vi "Format Channel Configuration Log.vi"(8 "error in (no error)":errorcluster, 10 "Channel Type (ao/ai)":enum16{"ao", "ai"}(ring), 11 "Instrument.Lockin in":refnum<class "Instrument.Lockin.lvclass">) -> (0 "error out":errorcluster, 1 "Channel Configuration":T1[](array[typedef]), 2 "Log Paths":string, 3 "Instrument.Lockin out":refnum<class "Instrument.Lockin.lvclass">, 4 "Times":timestamp[](array[timestamp]))   [LabVIEW 2019, in "Instrument.Lockin.lvlib" / "Instrument.Lockin.lvclass"]
uses:
  Instrument.Lockin.lvclass
  Typedefs/Lockin.LogConfiguration.Channels--Cluster.ctl
  Instrument.Lockin.lvclass/Instrument.Lockin.ctl
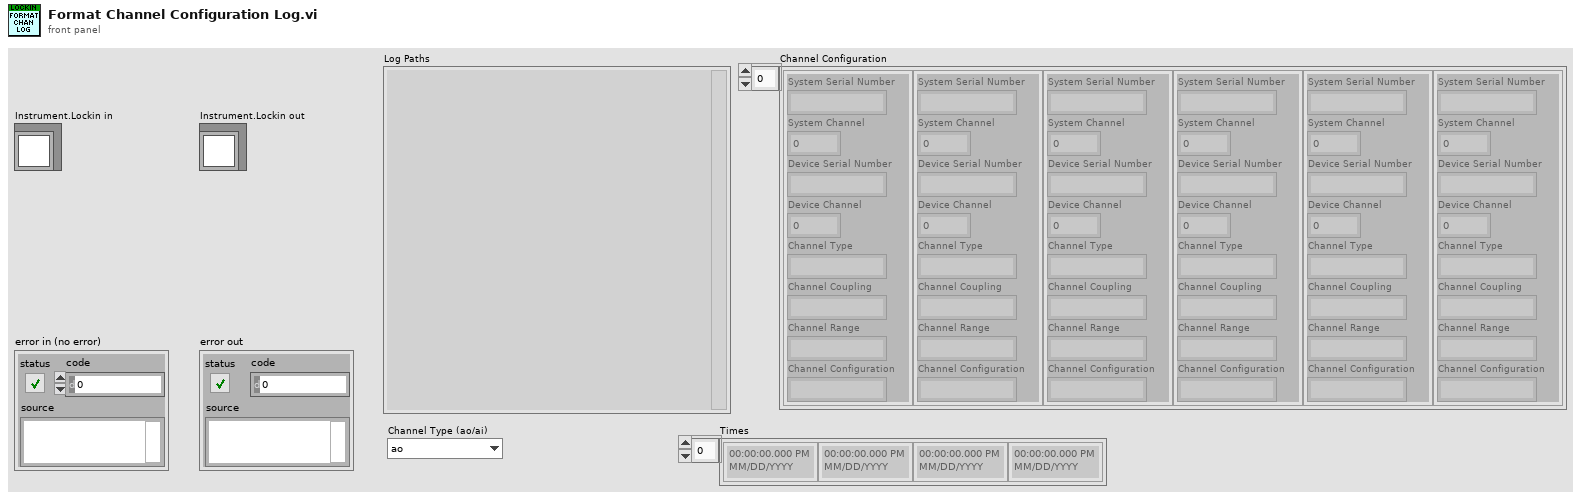
[diagram p1: front panel]
types:
  T1 = typedef "Instrument.Lockin.lvlib/Instrument.Lockin.lvclass/Lockin.LogConfiguration.Channels--Cluster.ctl" = cluster{"System Serial Number":string, "System Channel":i32, "Device Serial Number":string, "Device Channel":i32, "Channel Type":string, "Channel Coupling":string, "Channel Range":string, "Channel Configuration":string}
  T2 = typedef "Instrument.Lockin.lvlib/Instrument.DAQ.lvclass/AO.Channel--Cluster--Array.ctl" = T3[]
  T3 = typedef "Instrument.Lockin.lvlib/Instrument.DAQ.lvclass/AO.Channel--Cluster.ctl" = cluster{"Enable?":bool, "Channel":i32, "Amplitude":dbl, "Offset":dbl, "Frequency":dbl, "Phase":dbl, "Function":T4, "Sweeping?":bool, "Limit AC":bool, "Limit DC?":bool, "Duty Cycle":bool}
  T4 = typedef "Instrument.Lockin.lvlib/Instrument.DAQ.lvclass/AO.Channel.Function--Enum.ctl" = enum16{"sine", "square", "triangle", "saw"}
  T5 = typedef "Instrument.Lockin.lvlib/Instrument.DAQ.lvclass/DeviceInfo--Cluster.ctl" = cluster{"DeviceName":string, "DevIsSimulated":bool, "DeviceSerialNumber":string, "ProductType":string, "ProductCategory":i32, "ProductNumber":u32, "ChassisNumber":u32, "SlotNumber":u32, "ChassisName":string, "ChassisSerialNumber":string, "DevTemp":dbl, "SelfCal.LastDate/Time":string, "SelfCal.LastTemp":dbl, "calibration due?":bool}
  T6 = typedef "Instrument.Lockin.lvlib/Instrument.DAQ.lvclass/DAQ.Config.AO--Cluster--Array.ctl" = cluster{"Channels":tag, "Range":T7, "terminal configuration":T8, "Type":T9}[]
  T7 = typedef "Instrument.Lockin.lvlib/Instrument.DAQ.lvclass/DAQ.Config.AO.Range--enum.ctl" = enum16{"±0.1", "±1.0", "±10.0", ""}
  T8 = typedef "Instrument.Lockin.lvlib/Instrument.DAQ.lvclass/DAQ.TerminalConfiguration--ring.ctl" = i32
  T9 = typedef "Instrument.Lockin.lvlib/Instrument.DAQ.lvclass/DAQ.Type--enum.ctl" = enum16{"None", "USB-4431", "PXI-446x"}
  T10 = typedef "Instrument.Lockin.lvlib/Instrument.DAQ.lvclass/AI.Channel--Cluster--Array.ctl" = T11[]
  T11 = typedef "Instrument.Lockin.lvlib/Instrument.DAQ.lvclass/AI.Channel--Cluster.ctl" = cluster{"Enable?":bool, "Channel":i32, "References":u16[], "reference index":i32}
  T12 = typedef "Instrument.Lockin.lvlib/Instrument.DAQ.lvclass/DAQ.Config.AI--Cluster--Array.ctl" = cluster{"Channels":tag, "Coupling":T13, "Range":T14, "terminal configuration":T8, "Type":T9}[]
  T13 = typedef "Instrument.Lockin.lvlib/Instrument.DAQ.lvclass/DAQ.Config.AI.Coupling--enum.ctl" = u16
  T14 = typedef "Instrument.Lockin.lvlib/Instrument.DAQ.lvclass/DAQ.Config.AI.Range--enum.ctl" = enum16{"±0.316", "±1.00", "±3.16", "±10.0", "±31.6", "±42.4", ""}
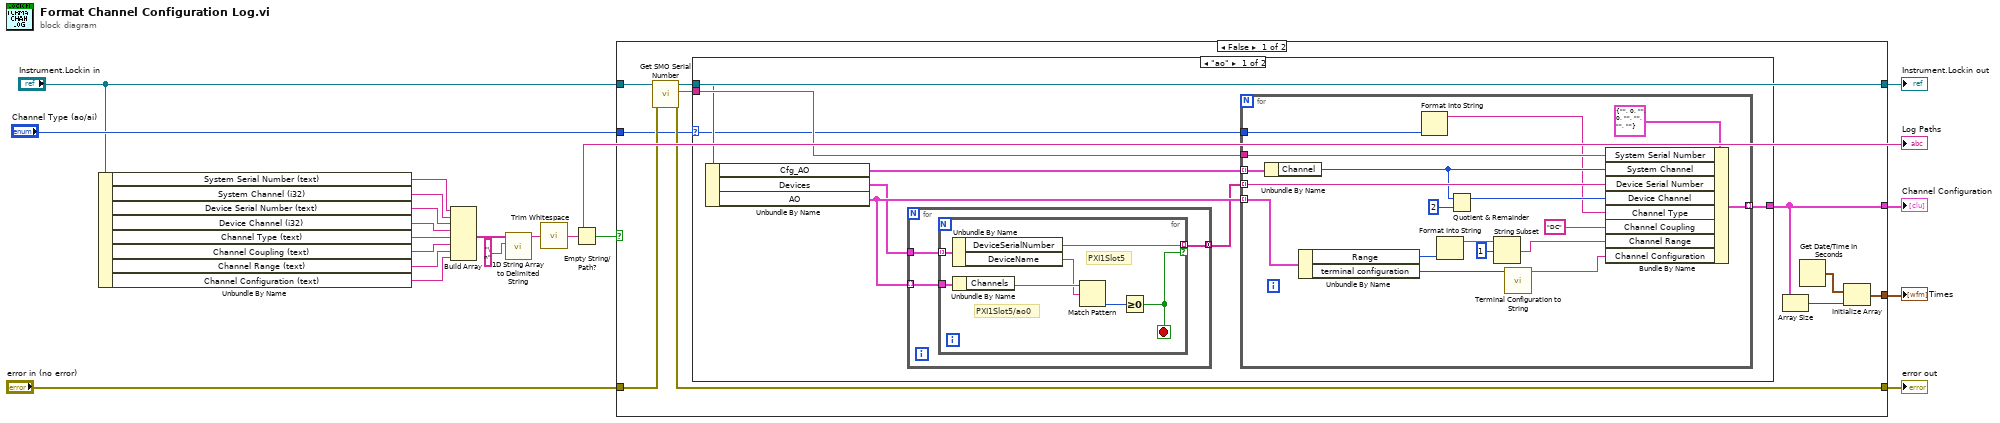
[diagram p0: block diagram]
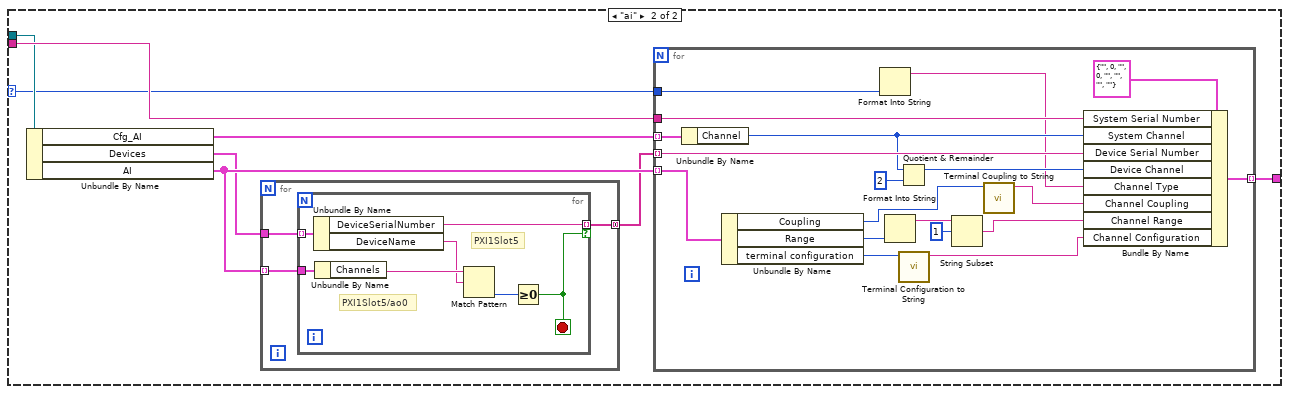
[diagram p2: hidden frame]
diagram:
  n1 = Unbundle By Name("Instrument.Lockin in") -> ("System Serial Number (text)"=w15:string, "System Channel (i32)"=w14:string, "Device Serial Number (text)"=w13:string, "Device Channel (i32)"=w12:string, "Channel Type (text)"=w11:string, "Channel Coupling (text)"=w10:string, "Channel Range (text)"=w9:string, "Channel Configuration (text)"=w8:string)
  n2 = Build Array(w15, w14, w13, w12, w11, w10, w9, w8) -> (w4:string[])
  n3 = call <vilib>:"1D String Array to Delimited String.vi"("delimiter"="\n", "string array"=w4) -> ("delimited string"=w5:string)  [unwired: 9 in]
  n4 = call <vilib>:"Trim Whitespace.vi"("string"=w5) -> ("trimmed string"=w2:string)  [unwired: 1 in]
  "Log Paths" <- w2
  n5 = Empty String/Path?(string/path=w2) -> (empty?=w3:bool)
  n6 = case shown="False" w3 {
    tunnel: "error in (no error)" -> [w29 w104]
    tunnel: [w28 w104] -> w19
    tunnel: [w27 w105] -> w18
    tunnel: [w22 _] -> w17
    tunnel: "Channel Type (ao/ai)" -> [w26 _]
    tunnel: "Instrument.Lockin in" -> [w25 w105]
    tunnel: [w21 _] -> w1
    frame False {
      n7 = call-dynamic "Get SMO Serial Number.vi"("error in (no error)"=w29, "Instrument.Lockin in"=w25) -> ("error out"=w28:errorcluster, "Serial Number"=w30:string, "Instrument.Lockin out"=w27:refnum<class "Instrument.Lockin.lvclass">)  [unwired: 7 in]
      n8 = case shown="\"ao\"" w26 {
        selector: w26 -> [w31 w67]
        tunnel: w30 -> [w38 w74]
        tunnel: w27 -> [w37 w73]
        tunnel: [w32 w68] -> w22
        frame "ao" {
          n9 = Unbundle By Name(w37) -> ("Cfg_AO"=w36:T2, "Devices"=w34:T5[], "AO"=w35:T6)
          n10 = for {
            tunnel: w34 -> [w41]
            tunnel: w35 -> [w40] mode=indexing
            tunnel: [w39] -> w33 mode=concatenating
            n11 = for {
              tunnel: w41 -> [w48] mode=indexing
              tunnel: w40 -> [w47]
              tunnel: [w43] -> w39 mode=indexing if=w42
              stop <- w42 stop-if-true
              # "PXI1Slot5"
              # "PXI1Slot5/ao0"
              n12 = Unbundle By Name(w48) -> ("DeviceSerialNumber"=w43:string, "DeviceName"=w45:string)
              n13 = Unbundle By Name(w47) -> ("Channels"=w46:tag)
              n14 = Match Pattern(string=w46, regular expression=w45) -> (offset past match=w44:i32)  [unwired: 1 in, 3 out]
              n15 = Greater Or Equal To 0?(x=w44) -> (x >= 0?=w42:bool)
            }
          }
          n16 = for {
            tunnel: [w66] -> w32 mode=indexing
            tunnel: w38 -> [w65]
            tunnel: w35 -> [w63] mode=indexing
            tunnel: w33 -> [w54] mode=indexing
            tunnel: w36 -> [w56] mode=indexing
            tunnel: w31 -> [w51]
            n17 = Unbundle By Name(w56) -> ("Channel"=w53:i32)
            n18 = Unbundle By Name(w63) -> ("Range"=w62:T7, "terminal configuration"=w50:T8)
            n19 = Format Into String(w51) -> (resulting string=w52:string)  [unwired: 3 in, 1 out]
            n20 = Format Into String(w62) -> (resulting string=w61:string)  [unwired: 3 in, 1 out]
            n21 = Quotient & Remainder(x=w53, y=2) -> (x-y*floor(x/y)=w58:i32)  [unwired: 1 out]
            n22 = String Subset(string=w61, offset (0)=1) -> (substring=w59:string)  [unwired: 1 in]
            n23 = call "Terminal Configuration to String.vi"("terminal configuration"=w50) -> ("f"=w49:string)  [unwired: 10 in]
            n24 = Bundle By Name(cluster=T1 {"System Serial Number"="", "System Channel"=0, "Device Serial Number"="", "Device Channel"=0, "Channel Type"="", "Channel Coupling"="", "Channel Range"="", "Channel Configuration"=""} ("DAQ Configuration"), "System Serial Number"=w65, "System Channel"=w53, "Device Serial Number"=w54, "Device Channel"=w58, "Channel Type"=w52, "Channel Coupling"="DC", "Channel Range"=w59, "Channel Configuration"=w49) -> (w66:T1)
          }
        }
        frame "ai" {
          n25 = Unbundle By Name(w73) -> ("Cfg_AI"=w72:T10, "Devices"=w70:T5[], "AI"=w71:T12)
          n26 = for {
            tunnel: w70 -> [w77]
            tunnel: w71 -> [w76] mode=indexing
            tunnel: [w75] -> w69 mode=concatenating
            n27 = for {
              tunnel: w77 -> [w84] mode=indexing
              tunnel: w76 -> [w83]
              tunnel: [w79] -> w75 mode=indexing if=w78
              stop <- w78 stop-if-true
              # "PXI1Slot5"
              # "PXI1Slot5/ao0"
              n28 = Unbundle By Name(w84) -> ("DeviceSerialNumber"=w79:string, "DeviceName"=w81:string)
              n29 = Unbundle By Name(w83) -> ("Channels"=w82:tag)
              n30 = Match Pattern(string=w82, regular expression=w81) -> (offset past match=w80:i32)  [unwired: 1 in, 3 out]
              n31 = Greater Or Equal To 0?(x=w80) -> (x >= 0?=w78:bool)
            }
          }
          n32 = for {
            tunnel: [w103] -> w68 mode=indexing
            tunnel: w74 -> [w102]
            tunnel: w71 -> [w100] mode=indexing
            tunnel: w69 -> [w92] mode=indexing
            tunnel: w72 -> [w93] mode=indexing
            tunnel: w67 -> [w89]
            n33 = Unbundle By Name(w93) -> ("Channel"=w91:i32)
            n34 = Unbundle By Name(w100) -> ("Coupling"=w85:T13, "Range"=w99:T14, "terminal configuration"=w87:T8)
            n35 = Format Into String(w89) -> (resulting string=w90:string)  [unwired: 3 in, 1 out]
            n36 = Format Into String(w99) -> (resulting string=w98:string)  [unwired: 3 in, 1 out]
            n37 = Quotient & Remainder(x=w91, y=2) -> (x-y*floor(x/y)=w95:i32)  [unwired: 1 out]
            n38 = call "Terminal Configuration to String.vi"("terminal configuration"=w87) -> ("f"=w88:string)  [unwired: 10 in]
            n39 = String Subset(string=w98, offset (0)=1) -> (substring=w96:string)  [unwired: 1 in]
            n40 = call "Terminal Coupling to String.vi"("Coupling"=w85) -> ("String"=w86:string)  [unwired: 10 in]
            n41 = Bundle By Name(cluster=T1 {"System Serial Number"="", "System Channel"=0, "Device Serial Number"="", "Device Channel"=0, "Channel Type"="", "Channel Coupling"="", "Channel Range"="", "Channel Configuration"=""} ("DAQ Configuration"), "System Serial Number"=w102, "System Channel"=w91, "Device Serial Number"=w92, "Device Channel"=w95, "Channel Type"=w90, "Channel Coupling"=w86, "Channel Range"=w96, "Channel Configuration"=w88) -> (w103:T1)
          }
        }
      }
      n42 = Array Size(array=w22) -> (size(s)=w24:i32)
      n43 = Get Date/Time In Seconds() -> (seconds since 1Jan1904=w23:timestamp)
      n44 = Initialize Array(w23, w24) -> (w21:timestamp[])
    }
    frame True {
    }
  }
  "Instrument.Lockin out" <- w18
  "error out" <- w19
  "Channel Configuration" <- w17
  "Times" <- w1
